vi "test-debouncer.vi"(8 "error in (no error)":errorcluster) -> (0 "error out":errorcluster, 3 "ALL TESTS PASSED":bool)   [LabVIEW 2019]
uses:
  <vilib>/Rock Robotics/WPI/ThirdParty/JAS_Junk/TrajLib/DEBOUNCER_TYPE_ENUM.ctl
  <vilib>/Rock Robotics/WPI/ThirdParty/JAS_Junk/TrajLib/Trajectory_Library.lvlib
panel:
  out "Test Passed 2":bool
  out "Test Passed 1":bool
  out "Test Passed 0":bool
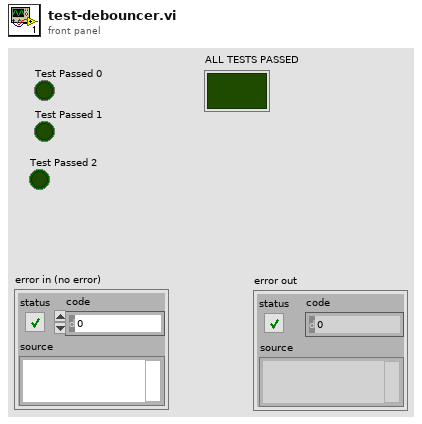
[diagram p1: front panel]
types:
  T1 = typedef "Trajectory_Library.lvlib/DEBOUNCER_TYPE_ENUM.ctl" = enum16{"Rising", "Falling", "Both"}
  T2 = typedef "Trajectory_Library.lvlib/DEBOUNCER.ctl" = cluster{"DebounceTimeSeconds":dbl, "PrevTimeSeconds":dbl, "Baseline":bool, "DebounceType":T1}
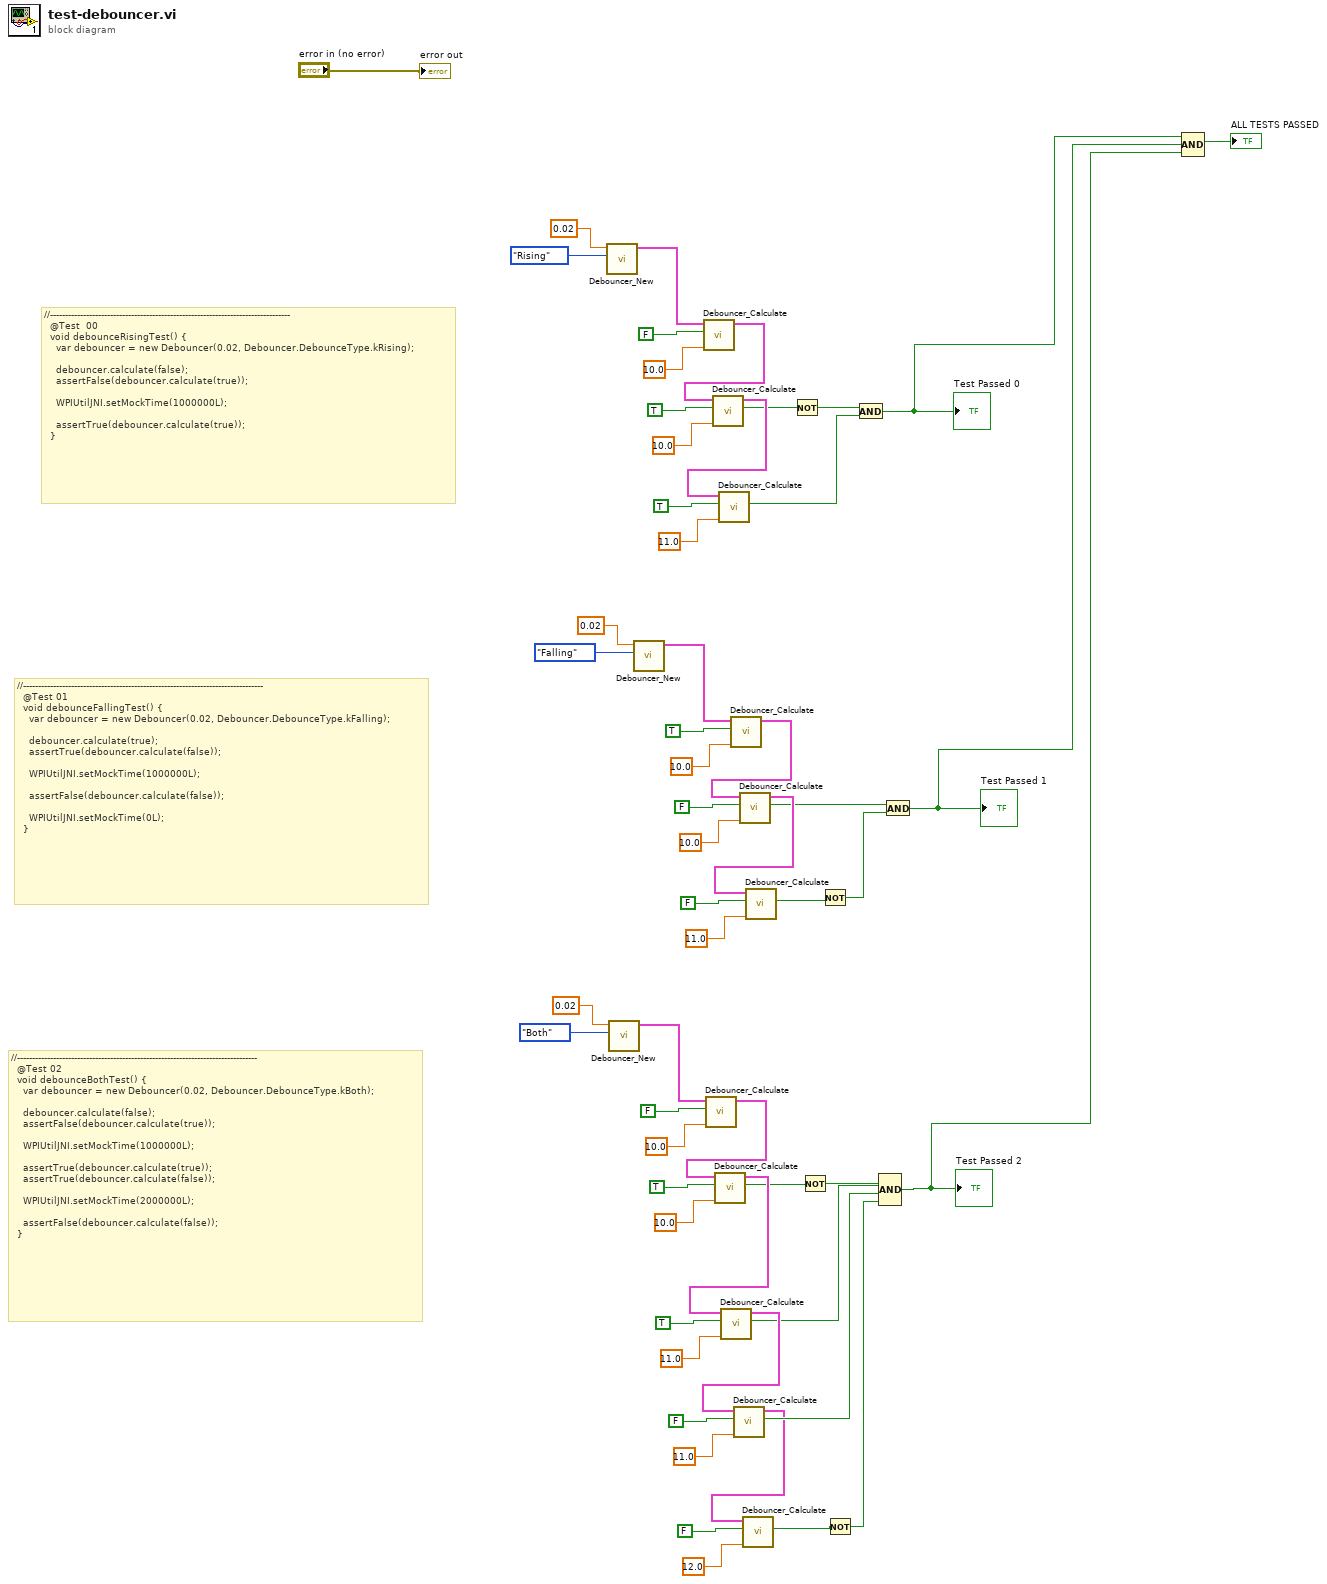
[diagram p0: block diagram]
diagram:
  # "//--------------------------------------------------------------------------------\n  @Test 02\n  void debounceBothTest() {\n    var debouncer = new Debouncer(0.02, Debouncer.DebounceType.kBoth);\n\n    debouncer.calculate(false);\n    assertFalse(debouncer.calculate(true));\n\n    WPIUtilJNI.setMockTime(1000000L);\n\n    assertTrue(debouncer.calculate(true));\n    assertTrue(debouncer.calculate(false));\n\n    WPIUtilJNI.setMockTime(2000000L);\n\n    assertFalse(debouncer.calculate(false));\n  }"
  # "//--------------------------------------------------------------------------------\n  @Test 01\n  void debounceFallingTest() {\n    var debouncer = new Debouncer(0.02, Debouncer.DebounceType.kFalling);\n\n    debouncer.calculate(true);\n    assertTrue(debouncer.calculate(false));\n\n    WPIUtilJNI.setMockTime(1000000L);\n\n    assertFalse(debouncer.calculate(false));\n\n    WPIUtilJNI.setMockTime(0L);\n  }"
  # "//--------------------------------------------------------------------------------\n  @Test  00\n  void debounceRisingTest() {\n    var debouncer = new Debouncer(0.02, Debouncer.DebounceType.kRising);\n\n    debouncer.calculate(false);\n    assertFalse(debouncer.calculate(true));\n\n    WPIUtilJNI.setMockTime(1000000L);\n\n    assertTrue(debouncer.calculate(true));\n  }"
  n1 = call <vilib>:"Debouncer_New.vi"("DebounceType"=DEBOUNCER_TYPE_ENUM."Rising", "DebounceTime"=0.02) -> ("Debouncer"=w53:T2)  [unwired: 8 in, 1 out]
  n2 = call <vilib>:"Debouncer_New.vi"("DebounceType"=DEBOUNCER_TYPE_ENUM."Both", "DebounceTime"=0.02) -> ("Debouncer"=w22:T2)  [unwired: 8 in, 1 out]
  n3 = call <vilib>:"Debouncer_New.vi"("DebounceType"=DEBOUNCER_TYPE_ENUM."Falling", "DebounceTime"=0.02) -> ("Debouncer"=w39:T2)  [unwired: 8 in, 1 out]
  n4 = call <vilib>:"Debouncer_Calculate.vi"("CurrentTIme"=10.0, "Input"=FALSE, "Debouncer In"=w53) -> ("Debouncer Out"=w46:T2)  [unwired: 6 in, 2 out]
  n5 = call <vilib>:"Debouncer_Calculate.vi"("CurrentTIme"=10.0, "Input"=FALSE, "Debouncer In"=w22) -> ("Debouncer Out"=w15:T2)  [unwired: 6 in, 2 out]
  n6 = call <vilib>:"Debouncer_Calculate.vi"("CurrentTIme"=10.0, "Input"=TRUE, "Debouncer In"=w46) -> ("Output"=w44:bool, "Debouncer Out"=w45:T2)  [unwired: 6 in, 1 out]
  n7 = call <vilib>:"Debouncer_Calculate.vi"("CurrentTIme"=10.0, "Input"=TRUE, "Debouncer In"=w15) -> ("Output"=w13:bool, "Debouncer Out"=w14:T2)  [unwired: 6 in, 1 out]
  n8 = call <vilib>:"Debouncer_Calculate.vi"("CurrentTIme"=11.0, "Input"=TRUE, "Debouncer In"=w45) -> ("Output"=w42:bool)  [unwired: 6 in, 2 out]
  n9 = call <vilib>:"Debouncer_Calculate.vi"("CurrentTIme"=11.0, "Input"=TRUE, "Debouncer In"=w14) -> ("Output"=w8:bool, "Debouncer Out"=w9:T2)  [unwired: 6 in, 1 out]
  n10 = call <vilib>:"Debouncer_Calculate.vi"("CurrentTIme"=10.0, "Input"=TRUE, "Debouncer In"=w39) -> ("Debouncer Out"=w32:T2)  [unwired: 6 in, 2 out]
  n11 = call <vilib>:"Debouncer_Calculate.vi"("CurrentTIme"=11.0, "Input"=FALSE, "Debouncer In"=w9) -> ("Output"=w7:bool, "Debouncer Out"=w4:T2)  [unwired: 6 in, 1 out]
  n12 = call <vilib>:"Debouncer_Calculate.vi"("CurrentTIme"=10.0, "Input"=FALSE, "Debouncer In"=w32) -> ("Output"=w30:bool, "Debouncer Out"=w31:T2)  [unwired: 6 in, 1 out]
  n13 = call <vilib>:"Debouncer_Calculate.vi"("CurrentTIme"=12.0, "Input"=FALSE, "Debouncer In"=w4) -> ("Output"=w3:bool)  [unwired: 6 in, 2 out]
  n14 = call <vilib>:"Debouncer_Calculate.vi"("CurrentTIme"=11.0, "Input"=FALSE, "Debouncer In"=w31) -> ("Output"=w29:bool)  [unwired: 6 in, 2 out]
  n15 = Not(x=w44) -> (.not. x?=w43:bool)
  n16 = Not(x=w13) -> (.not. x?=w12:bool)
  n17 = Not(x=w29) -> (.not. x?=w28:bool)
  n18 = Not(x=w3) -> (.not. x?=w2:bool)
  n19 = And(x=w43, y=w42) -> (x .and. y?=w26:bool)
  "Test Passed 0" <- w26
  n20 = Compound Arithmetic op=AND(w12, w8, w7, w2) -> (w1:bool)
  "Test Passed 2" <- w1
  n21 = And(x=w30, y=w28) -> (x .and. y?=w25:bool)
  "Test Passed 1" <- w25
  n22 = Compound Arithmetic op=AND(w26, w25, w1) -> (→"ALL TESTS PASSED":bool)
  "error out" <- "error in (no error)"
